vi "Icon Library.vi"(11 "Header Text":string) -> (1 "Class Wire Color":u32(colorbox), 2 "Private Data Icon":T1, 3 "Library Icon":T1)   [LabVIEW 2019, in "Builtins.lvlib"]
doc: "Creates the 8-bit icons for a LabVIEW Library (*.lvlib) or LabVIEW Class (*.lvclass) given the <b>Header Text</b>. The header background color is randomly generated.\n\nCreated by: Ryan Pacini"
uses:
  Builtins.lvlib
panel:
  out "data":picture
  out "header":picture
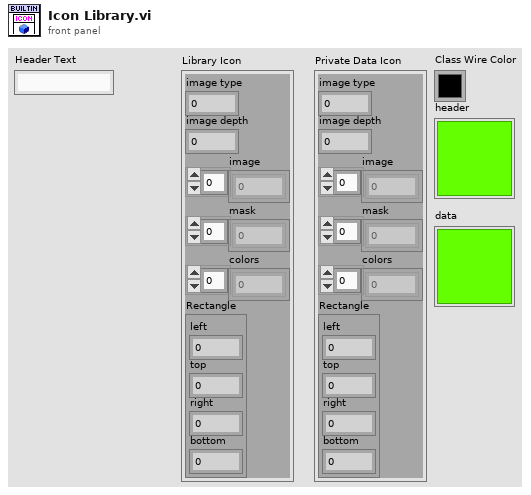
[diagram p1: front panel]
types:
  T1 = cluster{"image type":i32, "image depth":i32, "image":u8[], "mask":u8[], "colors":u32[], "Rectangle":cluster{"left":i16, "top":i16, "right":i16, "bottom":i16}}
  T2 = cluster{"left":i16, "top":i16, "right":i16, "bottom":i16}
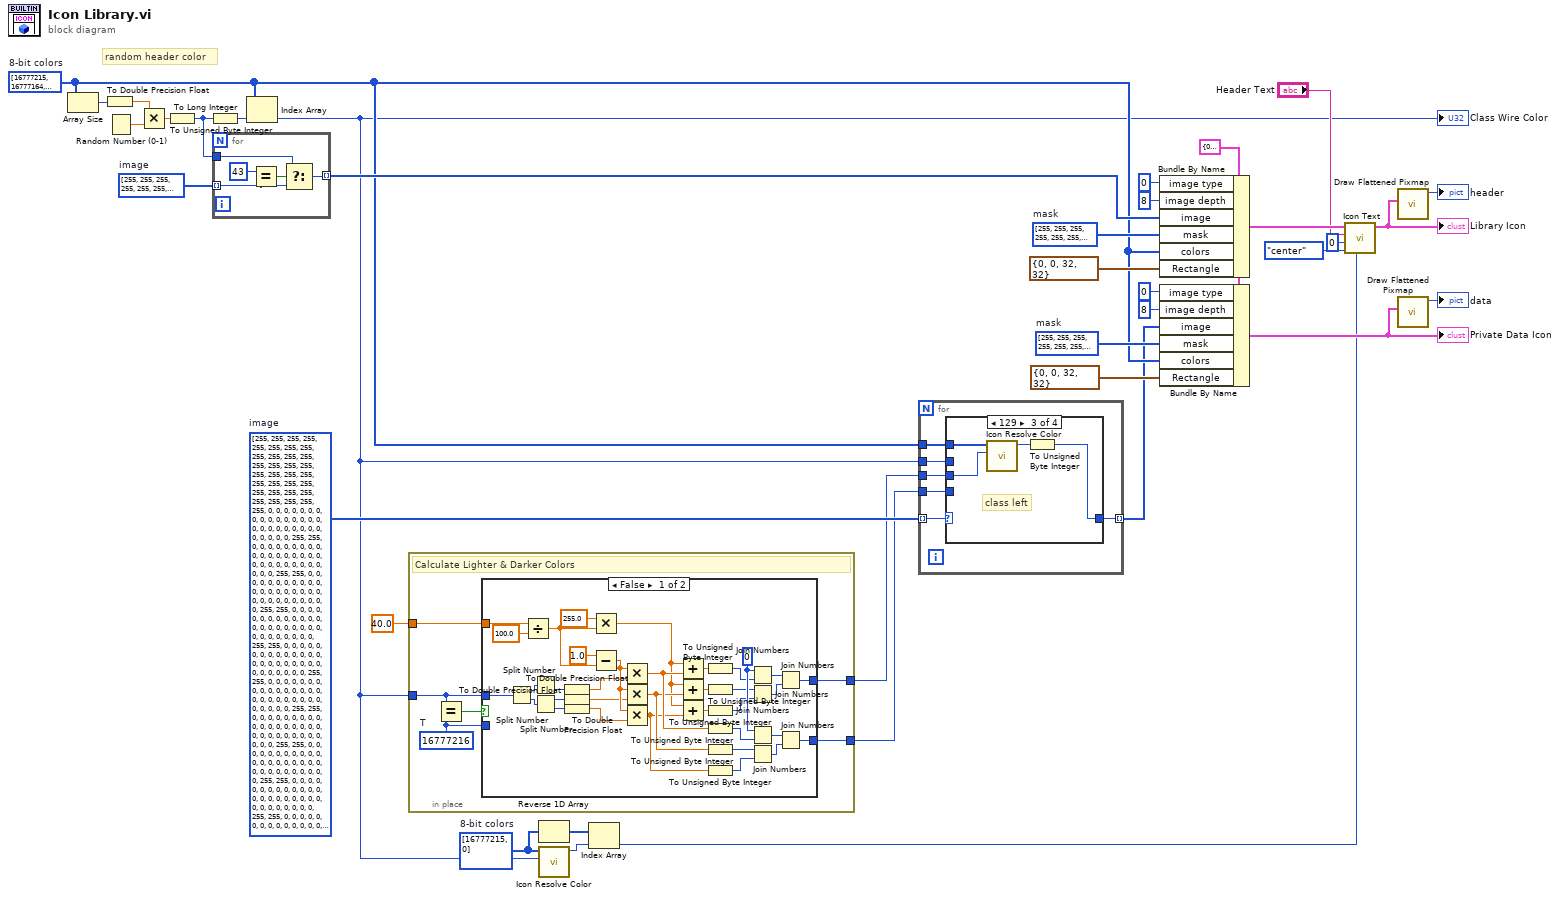
[diagram p0: block diagram]
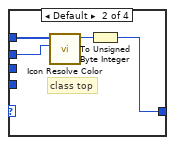
[diagram p4: hidden frame]
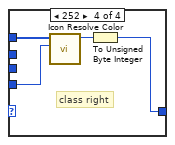
[diagram p5: hidden frame]
diagram:
  w4 = u32[] [16777215, 0]  # 8-bit colors
  w14 = u8[] [255, 255, 255, 255, 255, 255, 255, 255, 255, 255, 255, 255, 255, 255, 255, 255, 255, 255, 255, 255, 255, 255, 255, 255, 255, 255, 255, 255, 255, 255, 255, 255, 255, 0, 0, 0, 0, 0, 0, 0, 0, 0, 0, 0, 0, 0, 0, 0, 0, 0, 0, 0, 0, 0, 0, 0, 0, 0, 0, 0, 0, 0, 0, 255, 255, 0, 0, 0, 0, 0, 0, 0, 0, 0, 0, 0, 0, 0, 0, 0, 0, 0, 0, 0, 0, 0, 0, 0, 0, 0, 0, 0, 0, 0, 0, 255, 255, 0, 0, 0, 0, 0, 0, 0, 0, 0, 0, 0, 0, 0, 0, 0, 0, 0, 0, 0, 0, 0, 0, 0, 0, 0, 0, 0, 0, 0, 0, 255, 255, 0, 0, 0, 0, 0, 0, 0, 0, 0, 0, 0, 0, 0, 0, 0, 0, 0, 0, 0, 0, 0, 0, 0, 0, 0, 0, 0, 0, 0, 0, 255, 255, 0, 0, 0, 0, 0, 0, 0, 0, 0, 0, 0, 0, 0, 0, 0, 0, 0, 0, 0, 0, 0, 0, 0, 0, 0, 0, 0, 0, 0, 0, 255, 255, 0, 0, 0, 0, 0, 0, 0, 0, 0, 0, 0, 0, 0, 0, 0, 0, 0, 0, 0, 0, 0, 0, 0, 0, 0, 0, 0, 0, 0, 0, 255, 255, 0, 0, 0, 0, 0, 0, 0, 0, 0, 0, 0, 0, 0, 0, 0, 0, 0, 0, 0, 0, 0, 0, 0, 0, 0, 0, 0, 0, 0, 0, 255, 255, 0, 0, 0, 0, 0, 0, 0, 0, 0, 0, 0, 0, 0, 0, 0, 0, 0, 0, 0, 0, 0, 0, 0, 0, 0, 0, 0, 0, 0, 0, 255, 255, 0, 0, 0, 0, 0, 0, 0, 0, 0, 0, 0, 0, 0, 0, 0, 0, 0, 0, 0, 0, 0, 0, 0, 0, 0, 0, 0, 0, 0, 0, 255, 255, 0, 0, 0, 0, 0, 0, 0, 0, 0, 0, 0, 0, 0, 0, 0, 0, 0, 0, 0, 0, 0, 0, 0, 0, 0, 0, 0, 0, 0, 0, 255, 255, 0, 0, 0, 0, 0, 0, 0, 0, 0, 0, 0, 0, 0, 0, 172, 172, 0, 0, 0, 0, 0, 0, 0, 0, 0, 0, 0, 0, 0, 0, 255, 255, 0, 0, 0, 0, 0, 0, 0, 0, 0, 0, 0, 0, 172, 172, 86, 86, 172, 172, 0, 0, 0, 0, 0, 0, 0, 0, 0, 0, 0, 0, 255, 255, 0, 0, 0, 0, 0, 0, 0, 0, 0, 0, 172, 172, 86, 86, 86, 86, 86, 86, 172, 172, 0, 0, 0, 0, 0, 0, 0, 0, 0, 0, 255, 255, 0, 0, 0, 0, 0, 0, 0, 0, 172, 172, 86, 86, 86, 86, 86, 86, 86, 86, 86, 86, 172, 172, 0, 0, 0, 0, 0, 0, 0, 0, 255, 255, 0, 0, 0, 0, 0, 0, 0, 172, 86, 86, 86, 86, 86, 86, 86, 86, 86, 86, 86, 86, 86, 86, 252, 0, 0, 0, 0, 0, 0, 0, 255, 255, 0, 0, 0, 0, 0, 0, 0, 129, 129, 86, 86, 86, 86, 86, 86, 86, 86, 86, 86, 86, 86, 252, 252, 0, 0, 0, 0, 0, 0, 0, 255, 255, 0, 0, 0, 0, 0, 0, 0, 129, 129, 129, 129, 86, 86, 86, 86, 86, 86, 86, 86, 252, 252, 252, 252, 0, 0, 0, 0, 0, 0, 0, 255, 255, 0, 0, 0, 0, 0, 0, 0, 129, 129, 129, 129, 129, 129, 86, 86, 86, 86, 252, 252, 252, 252, 252, 252, 0, 0, 0, 0, 0, 0, 0, 255, 255, 0, 0, 0, 0, 0, 0, 0, 129, 129, 129, 129, 129, 129, 129, 129, 252, 252, 252, 252, 252, 252, 252, 252, 0, 0, 0, 0, 0, 0, 0, 255, 255, 0, 0, 0, 0, 0, 0, 0, 129, 129, 129, 129, 129, 129, 129, 129, 252, 252, 252, 252, 252, 252, 252, 252, 0, 0, 0, 0, 0, 0, 0, 255, 255, 0, 0, 0, 0, 0, 0, 0, 129, 129, 129, 129, 129, 129, 129, 129, 252, 252, 252, 252, 252, 252, 252, 252, 0, 0, 0, 0, 0, 0, 0, 255, 255, 0, 0, 0, 0, 0, 0, 0, 129, 129, 129, 129, 129, 129, 129, 129, 252, 252, 252, 252, 252, 252, 252, 252, 0, 0, 0, 0, 0, 0, 0, 255, 255, 0, 0, 0, 0, 0, 0, 0, 129, 129, 129, 129, 129, 129, 129, 129, 252, 252, 252, 252, 252, 252, 252, 252, 0, 0, 0, 0, 0, 0, 0, 255, 255, 0, 0, 0, 0, 0, 0, 0, 129, 129, 129, 129, 129, 129, 129, 129, 252, 252, 252, 252, 252, 252, 252, 252, 0, 0, 0, 0, 0, 0, 0, 255, 255, 0, 0, 0, 0, 0, 0, 0, 129, 129, 129, 129, 129, 129, 129, 129, 252, 252, 252, 252, 252, 252, 252, 252, 0, 0, 0, 0, 0, 0, 0, 255, 255, 0, 0, 0, 0, 0, 0, 0, 0, 129, 129, 129, 129, 129, 129, 129, 252, 252, 252, 252, 252, 252, 252, 0, 0, 0, 0, 0, 0, 0, 0, 255, 255, 0, 0, 0, 0, 0, 0, 0, 0, 0, 0, 129, 129, 129, 129, 129, 252, 252, 252, 252, 252, 0, 0, 0, 0, 0, 0, 0, 0, 0, 0, 255, 255, 0, 0, 0, 0, 0, 0, 0, 0, 0, 0, 0, 0, 129, 129, 129, 252, 252, 252, 0, 0, 0, 0, 0, 0, 0, 0, 0, 0, 0, 0, 255, 255, 0, 0, 0, 0, 0, 0, 0, 0, 0, 0, 0, 0, 0, 0, 129, 252, 0, 0, 0, 0, 0, 0, 0, 0, 0, 0, 0, 0, 0, 0, 255, 255, 0, 0, 0, 0, 0, 0, 0, 0, 0, 0, 0, 0, 0, 0, 0, 0, 0, 0, 0, 0, 0, 0, 0, 0, 0, 0, 0, 0, 0, 0, 255, 255, 255, 255, 255, 255, 255, 255, 255, 255, 255, 255, 255, 255, 255, 255, 255, 255, 255, 255, 255, 255, 255, 255, 255, 255, 255, 255, 255, 255, 255, 255, 255]  # image
  w23 = u8[] [255, 255, 255, 255, 255, 255, 255, 255, 255, 255, 255, 255, 255, 255, 255, 255, 255, 255, 255, 255, 255, 255, 255, 255, 255, 255, 255, 255, 255, 255, 255, 255, 255, 255, 255, 255, 255, 255, 255, 255, 255, 255, 255, 255, 255, 255, 255, 255, 255, 255, 255, 255, 255, 255, 255, 255, 255, 255, 255, 255, 255, 255, 255, 255, 255, 255, 255, 255, 255, 255, 255, 255, 255, 255, 255, 255, 255, 255, 255, 255, 255, 255, 255, 255, 255, 255, 255, 255, 255, 255, 255, 255, 255, 255, 255, 255, 255, 255, 255, 255, 255, 255, 255, 255, 255, 255, 255, 255, 255, 255, 255, 255, 255, 255, 255, 255, 255, 255, 255, 255, 255, 255, 255, 255, 255, 255, 255, 255]  # mask
  w30 = u8[] [255, 255, 255, 255, 255, 255, 255, 255, 255, 255, 255, 255, 255, 255, 255, 255, 255, 255, 255, 255, 255, 255, 255, 255, 255, 255, 255, 255, 255, 255, 255, 255, 255, 255, 255, 255, 0, 0, 0, 0, 0, 0, 0, 0, 0, 0, 0, 0, 0, 0, 0, 0, 0, 0, 0, 0, 0, 0, 0, 0, 0, 0, 0, 0, 0, 0, 0, 0, 0, 0, 0, 0, 0, 0, 0, 0, 0, 0, 0, 0, 0, 0, 0, 0, 0, 0, 0, 0, 0, 0, 0, 0, 0, 0, 0, 0, 0, 0, 0, 0, 0, 0, 0, 0, 0, 0, 0, 0, 0, 0, 0, 0, 0, 0, 0, 0, 0, 0, 0, 0, 0, 0, 0, 0, 0, 0, 0, 0]  # mask
  w22 = T1 {"image type"=0, "image depth"=0, "image"=[], "mask"=[], "colors"=[], "Rectangle"={"left"=0, "top"=0, "right"=0, "bottom"=0}} ("image data")
  w33 = u8[] [255, 255, 255, 255, 255, 255, 255, 255, 255, 255, 255, 255, 255, 255, 255, 255, 255, 255, 255, 255, 255, 255, 255, 255, 255, 255, 255, 255, 255, 255, 255, 255, 255, 43, 43, 43, 43, 43, 43, 43, 43, 43, 43, 43, 43, 43, 43, 43, 43, 43, 43, 43, 43, 43, 43, 43, 43, 43, 43, 43, 43, 43, 43, 255, 255, 43, 43, 43, 43, 43, 43, 43, 43, 43, 43, 43, 43, 43, 43, 43, 43, 43, 43, 43, 43, 43, 43, 43, 43, 43, 43, 43, 43, 43, 43, 255, 255, 43, 43, 43, 43, 43, 43, 43, 43, 43, 43, 43, 43, 43, 43, 43, 43, 43, 43, 43, 43, 43, 43, 43, 43, 43, 43, 43, 43, 43, 43, 255, 255, 43, 43, 43, 43, 43, 43, 43, 43, 43, 43, 43, 43, 43, 43, 43, 43, 43, 43, 43, 43, 43, 43, 43, 43, 43, 43, 43, 43, 43, 43, 255, 255, 43, 43, 43, 43, 43, 43, 43, 43, 43, 43, 43, 43, 43, 43, 43, 43, 43, 43, 43, 43, 43, 43, 43, 43, 43, 43, 43, 43, 43, 43, 255, 255, 43, 43, 43, 43, 43, 43, 43, 43, 43, 43, 43, 43, 43, 43, 43, 43, 43, 43, 43, 43, 43, 43, 43, 43, 43, 43, 43, 43, 43, 43, 255, 255, 43, 43, 43, 43, 43, 43, 43, 43, 43, 43, 43, 43, 43, 43, 43, 43, 43, 43, 43, 43, 43, 43, 43, 43, 43, 43, 43, 43, 43, 43, 255, 255, 255, 255, 255, 255, 255, 255, 255, 255, 255, 255, 255, 255, 255, 255, 255, 255, 255, 255, 255, 255, 255, 255, 255, 255, 255, 255, 255, 255, 255, 255, 255, 0, 0, 0, 0, 0, 0, 0, 0, 0, 0, 0, 0, 0, 0, 0, 0, 0, 0, 0, 0, 0, 0, 0, 0, 0, 0, 0, 0, 0, 0, 0, 0, 0, 0, 0, 0, 0, 0, 0, 0, 0, 0, 0, 0, 0, 0, 0, 0, 0, 0, 0, 0, 0, 0, 0, 0, 0, 0, 0, 0, 0, 0, 0, 0, 0, 0, 0, 0, 0, 0, 0, 0, 0, 0, 0, 0, 0, 0, 0, 0, 0, 0, 0, 0, 0, 0, 0, 0, 0, 0, 0, 0, 0, 0, 0, 0, 0, 0, 0, 0, 0, 0, 0, 0, 0, 0, 0, 0, 0, 0, 0, 0, 0, 0, 0, 0, 0, 0, 0, 0, 0, 0, 0, 0, 0, 0, 0, 0, 0, 0, 0, 0, 0, 0, 0, 0, 0, 0, 0, 0, 0, 0, 0, 0, 0, 0, 0, 0, 0, 0, 0, 0, 0, 0, 0, 0, 0, 0, 0, 0, 0, 0, 0, 0, 0, 0, 0, 0, 0, 0, 0, 0, 0, 0, 0, 0, 0, 0, 0, 0, 0, 0, 0, 0, 0, 0, 0, 0, 0, 0, 0, 0, 0, 0, 0, 0, 0, 0, 0, 0, 0, 0, 0, 0, 0, 0, 0, 0, 0, 0, 0, 0, 0, 0, 0, 0, 0, 0, 0, 0, 0, 0, 0, 0, 0, 0, 0, 0, 0, 0, 0, 0, 0, 0, 0, 0, 0, 0, 0, 0, 0, 0, 0, 0, 0, 0, 0, 0, 0, 0, 0, 0, 0, 0, 0, 0, 0, 0, 0, 0, 0, 0, 0, 0, 0, 0, 0, 0, 0, 0, 0, 0, 0, 0, 0, 0, 0, 0, 0, 0, 0, 0, 0, 0, 0, 0, 0, 0, 0, 0, 0, 0, 0, 0, 0, 0, 0, 0, 0, 0, 0, 0, 0, 0, 0, 0, 0, 0, 0, 0, 0, 0, 0, 0, 0, 0, 0, 0, 0, 0, 0, 0, 0, 0, 0, 0, 0, 0, 0, 0, 0, 0, 0, 0, 0, 0, 0, 0, 0, 0, 0, 0, 0, 0, 0, 0, 0, 0, 0, 0, 0, 0, 0, 0, 0, 0, 0, 0, 0, 0, 0, 0, 0, 0, 0, 0, 0, 0, 0, 0, 0, 0, 0, 0, 0, 0, 0, 0, 0, 0, 0, 0, 0, 0, 0, 0, 0, 0, 0, 0, 0, 0, 0, 0, 0, 0, 0, 0, 0, 0, 0, 0, 0, 0, 0, 0, 0, 0, 0, 0, 0, 0, 0, 0, 0, 0, 0, 0, 0, 0, 0, 0, 0, 0, 0, 0, 0, 0, 0, 0, 0, 0, 0, 0, 0, 0, 0, 0, 0, 0, 0, 0, 0, 0, 0, 0, 0, 0, 0, 0, 0, 0, 0, 0, 0, 0, 0, 0, 0, 0, 0, 0, 0, 0, 0, 0, 0, 0, 0, 0, 0, 0, 0, 0, 0, 0, 0, 0, 0, 0, 0, 0, 0, 0, 0, 0, 0, 0, 0, 0, 0, 0, 0, 0, 0, 0, 0, 0, 0, 0, 0, 0, 0, 0, 0, 0, 0, 0, 0, 0, 0, 0, 0, 0, 0, 0, 0, 0, 0, 0, 0, 0, 0, 0, 0, 0, 0, 0, 0, 0, 0, 0, 0, 0, 0, 0, 0, 0, 0, 0, 0, 0, 0, 0, 0, 0, 0, 0, 0, 0, 0, 0, 0, 0, 0, 0, 0, 0, 0, 0, 0, 0, 0, 0, 0, 0, 0, 0, 0, 0, 0, 0, 0, 0, 0, 0, 0, 0, 0, 0, 0, 0, 0, 0, 0, 0, 0, 0, 0, 0, 0, 0, 0, 0, 0, 0, 0, 0, 0, 0, 0, 0, 0, 0, 0, 0, 0, 0, 0, 0, 0, 0, 0, 0, 0, 0, 0, 0, 0, 0, 0, 0, 0, 0, 0, 0, 0, 0, 0, 0, 0, 0, 0, 0, 0, 0, 0, 0, 0, 0, 0, 0, 0, 0, 0, 0, 0, 0, 0, 0, 0, 0, 0, 0, 0, 0, 0, 0, 0, 0, 0, 0, 0, 0, 0, 0, 0, 0, 0, 0, 0, 0, 0, 0, 0, 0, 0, 0, 0, 0, 0, 0, 0, 0, 0, 0, 0, 0, 0, 0, 0, 0, 0, 0, 0, 0, 0, 0, 0, 0, 0, 0, 0, 0, 0, 0, 0, 0, 0, 0, 0, 0, 0, 0, 0, 0, 0, 0, 0, 0, 0, 0, 0, 0, 0, 0, 0, 0, 0, 0, 0, 0, 0, 0, 0, 0]  # image
  w16 = u32[] [16777215, 16777164, 16777113, 16777062, 16777011, 16776960, 16764159, 16764108, 16764057, 16764006, 16763955, 16763904, 16751103, 16751052, 16751001, 16750950, 16750899, 16750848, 16738047, 16737996, 16737945, 16737894, 16737843, 16737792, 16724991, 16724940, 16724889, 16724838, 16724787, 16724736, 16711935, 16711884, 16711833, 16711782, 16711731, 16711680, 13434879, 13434828, 13434777, 13434726, 13434675, 13434624, 13421823, 13421772, 13421721, 13421670, 13421619, 13421568, 13408767, 13408716, 13408665, 13408614, 13408563, 13408512, 13395711, 13395660, 13395609, 13395558, 13395507, 13395456, 13382655, 13382604, 13382553, 13382502, 13382451, 13382400, 13369599, 13369548, 13369497, 13369446, 13369395, 13369344, 10092543, 10092492, 10092441, 10092390, 10092339, 10092288, 10079487, 10079436, 10079385, 10079334, 10079283, 10079232, 10066431, 10066380, 10066329, 10066278, 10066227, 10066176, 10053375, 10053324, 10053273, 10053222, 10053171, 10053120, 10040319, 10040268, 10040217, 10040166, 10040115, 10040064, 10027263, 10027212, 10027161, 10027110, 10027059, 10027008, 6750207, 6750156, 6750105, 6750054, 6750003, 6749952, 6737151, 6737100, 6737049, 6736998, 6736947, 6736896, 6724095, 6724044, 6723993, 6723942, 6723891, 6723840, 6711039, 6710988, 6710937, 6710886, 6710835, 6710784, 6697983, 6697932, 6697881, 6697830, 6697779, 6697728, 6684927, 6684876, 6684825, 6684774, 6684723, 6684672, 3407871, 3407820, 3407769, 3407718, 3407667, 3407616, 3394815, 3394764, 3394713, 3394662, 3394611, 3394560, 3381759, 3381708, 3381657, 3381606, 3381555, 3381504, 3368703, 3368652, 3368601, 3368550, 3368499, 3368448, 3355647, 3355596, 3355545, 3355494, 3355443, 3355392, 3342591, 3342540, 3342489, 3342438, 3342387, 3342336, 65535, 65484, 65433, 65382, 65331, 65280, 52479, 52428, 52377, 52326, 52275, 52224, 39423, 39372, 39321, 39270, 39219, 39168, 26367, 26316, 26265, 26214, 26163, 26112, 13311, 13260, 13209, 13158, 13107, 13056, 255, 204, 153, 102, 51, 15597568, 14483456, 12255232, 11141120, 8912896, 7798784, 5570560, 4456448, 2228224, 1114112, 60928, 56576, 47872, 43520, 34816, 30464, 21760, 17408, 8704, 4352, 238, 221, 187, 170, 136, 119, 85, 68, 34, 17, 15658734, 14540253, 12303291, 11184810, 8947848, 7829367, 5592405, 4473924, 2236962, 1118481, 0]  # 8-bit colors
  # "random header color"
  n1 = Array Size(array=w16) -> (size(s)=w20:i32)
  n2 = To Double Precision Float(number=w20) -> (double precision float=w18:dbl)
  n3 = Random Number (0-1)() -> (number: 0 to 1=w19:dbl)
  n4 = Multiply(x=w18, y=w19) -> (x*y=w17:dbl)
  n5 = To Unsigned Byte Integer(number=w17) -> (unsigned 8bit integer=w31:u8)
  n6 = To Long Integer(number=w31) -> (32bit integer=w32:i32)
  n7 = for {
    tunnel: [w41] -> w29 mode=indexing
    tunnel: w33 -> [w40] mode=indexing
    tunnel: w31 -> [w37]
    n8 = Equal?(x=u8 43, y=w40) -> (x = y?=w38:bool)
    n9 = Select(t=w37, s=w38, f=w40) -> (s? t:f=w41:u8)
  }
  n10 = Index Array(array=w16, index=w32) -> (element=w5:u32)
  "Class Wire Color" <- w5
  n11 = in-place {
    in-place-border: 40.0 ("Percentage(30)") -> [w47]
    in-place-border: w5 -> [w46]
    in-place-border: [w45] -> w12
    in-place-border: [w44] -> w11
    w42 = u32 16777216  # T
    # "Calculate Lighter & Darker Colors"
    n12 = Equal?(x=w46, y=w42) -> (x = y?=w43:bool)
    n13 = case shown="False" w43 {
      tunnel: [w55 w83] -> w44
      tunnel: [w54 w83] -> w45
      tunnel: w46 -> [w82 _]
      tunnel: w42 -> [_ w83]
      tunnel: w47 -> [w56 _]
      frame False {
        w69 = u8 0
        n14 = Split Number(x=w82) -> (hi(x)=w57:u16, lo(x)=w58:u16)
        n15 = Divide(x=w56, y=100.0) -> (x/y=w81:dbl)
        n16 = Split Number(x=w57) -> (lo(x)=w80:u8)  [unwired: 1 out]
        n17 = Split Number(x=w58) -> (hi(x)=w79:u8, lo(x)=w78:u8)
        n18 = To Double Precision Float(number=w80) -> (double precision float=w50:dbl)
        n19 = To Double Precision Float(number=w79) -> (double precision float=w49:dbl)
        n20 = To Double Precision Float(number=w78) -> (double precision float=w48:dbl)
        n21 = Multiply(x=255.0, y=w81) -> (x*y=w73:dbl)
        n22 = Subtract(x=1.0, y=w81) -> (x-y=w77:dbl)
        n23 = Multiply(x=w77, y=w50) -> (x*y=w76:dbl)
        n24 = Multiply(x=w77, y=w49) -> (x*y=w75:dbl)
        n25 = Multiply(x=w77, y=w48) -> (x*y=w74:dbl)
        n26 = Add(x=w73, y=w76) -> (x+y=w72:dbl)
        n27 = Add(x=w73, y=w75) -> (x+y=w71:dbl)
        n28 = Add(x=w73, y=w74) -> (x+y=w70:dbl)
        n29 = To Unsigned Byte Integer(number=w72) -> (unsigned 8bit integer=w68:u8)
        n30 = To Unsigned Byte Integer(number=w71) -> (unsigned 8bit integer=w67:u8)
        n31 = To Unsigned Byte Integer(number=w70) -> (unsigned 8bit integer=w66:u8)
        n32 = To Unsigned Byte Integer(number=w76) -> (unsigned 8bit integer=w59:u8)
        n33 = To Unsigned Byte Integer(number=w75) -> (unsigned 8bit integer=w60:u8)
        n34 = To Unsigned Byte Integer(number=w74) -> (unsigned 8bit integer=w61:u8)
        n35 = Join Numbers(hi=w69, lo=w68) -> ((hi.lo)=w64:u16)
        n36 = Join Numbers(hi=w67, lo=w66) -> ((hi.lo)=w65:u16)
        n37 = Join Numbers(hi=w69, lo=w59) -> ((hi.lo)=w62:u16)
        n38 = Join Numbers(hi=w60, lo=w61) -> ((hi.lo)=w63:u16)
        n39 = Join Numbers(hi=w64, lo=w65) -> ((hi.lo)=w54:u32)
        n40 = Join Numbers(hi=w62, lo=w63) -> ((hi.lo)=w55:u32)
      }
      frame True {
      }
    }
  }
  n41 = Reverse 1D Array(array=w4) -> (reversed array=w3:u32[])
  n42 = call "Icon Resolve Color.vi"("color"=w5, "8-bit colors"=w4) -> ("index"=w2:i32)  [unwired: 8 in, 1 out]
  n43 = Index Array(array=w3, index=w2) -> (element=w1:u32)
  n44 = for {
    tunnel: w14 -> [w89] mode=indexing
    tunnel: w5 -> [w88]
    tunnel: [w87] -> w15 mode=indexing
    tunnel: w16 -> [w86]
    tunnel: w12 -> [w85]
    tunnel: w11 -> [w84]
    n45 = case shown="129" w89 {
      selector: w89 -> [w90 _ _ _]
      tunnel: w88 -> [_ w91 _ _]
      tunnel: [w90 w92 w96 w100] -> w87
      tunnel: w86 -> [_ w94 w98 w102]
      tunnel: w85 -> [_ _ w95 _]
      tunnel: w84 -> [_ _ _ w99]
      frame 0, 255 {
        # "border"
      }
      frame Default {
        # "class top"
        n46 = call "Icon Resolve Color.vi"("color"=w91, "8-bit colors"=w94) -> ("index"=w93:i32)  [unwired: 8 in, 1 out]
        n47 = To Unsigned Byte Integer(number=w93) -> (unsigned 8bit integer=w92:u8)
      }
      frame 129 {
        # "class left"
        n48 = call "Icon Resolve Color.vi"("color"=w95, "8-bit colors"=w98) -> ("index"=w97:i32)  [unwired: 8 in, 1 out]
        n49 = To Unsigned Byte Integer(number=w97) -> (unsigned 8bit integer=w96:u8)
      }
      frame 252 {
        # "class right"
        n50 = call "Icon Resolve Color.vi"("color"=w99, "8-bit colors"=w102) -> ("index"=w101:i32)  [unwired: 8 in, 1 out]
        n51 = To Unsigned Byte Integer(number=w101) -> (unsigned 8bit integer=w100:u8)
      }
    }
  }
  n52 = Bundle By Name(cluster=w22, "image type"=0, "image depth"=8, "image"=w29, "mask"=w30, "colors"=w16, "Rectangle"=T2 {"left"=0, "top"=0, "right"=32, "bottom"=32}) -> (w10:T1)
  n53 = Bundle By Name(cluster=w22, "image type"=0, "image depth"=8, "image"=w15, "mask"=w23, "colors"=w16, "Rectangle"=T2 {"left"=0, "top"=0, "right"=32, "bottom"=32}) -> (w34:T1)
  "Private Data Icon" <- w34
  n54 = call "Icon Text.vi"("Text Color (Black)"=w1, "Justify (center)"=enum8{"center", "left", "right"}."center", "Top (0)"=0, "Text"="Header Text", "Image in"=w10) -> ("Image out"=w9:T1)  [unwired: 6 in]
  "Library Icon" <- w9
  n55 = call <vilib>:"Draw Flattened Pixmap.vi"("image data"=w9) -> ("new picture"=→"header":picture)  [unwired: 8 in]
  n56 = call <vilib>:"Draw Flattened Pixmap.vi"("image data"=w34) -> ("new picture"=→"data":picture)  [unwired: 8 in]
